vi "TestingThingsWithRobotSimulator.vi"() -> ()   [LabVIEW 2016]
uses:
  <vilib>/addons/control/pid/pid.llb/PID (DBL).vi
  <vilib>/addons/control/pid/NI_PID_pid.lvlib
panel:
  in  "Radius":dbl=200.0
  out "AngleVel":cluster{dbl, dbl}(graph)={199.99833333333333, 200.08337175954182}
  out "AnglePos":cluster{dbl, dbl}(graph)={199.99833333333333, 200.08337175954182}
  in  "Angular Constants":T1={"FF"=0.0085, "PID gains"={"P"=0.1, "I"=0.0, "D"=0.0}} {"PID gains"."D" format="%.5f"; "PID gains"."I" format="%.3f"; "PID gains"."P" format="%.3f"}
  out "Position":cluster{dbl, dbl}(graph)={199.99833333333333, 200.08337175954182}
  in  "Linear Constants":T1={"FF"=0.0085, "PID gains"={"P"=0.1, "I"=0.0, "D"=0.0}} {"PID gains"."D" format="%.5f"; "PID gains"."I" format="%.3f"; "PID gains"."P" format="%.3f"}
  out "Velocity":cluster{dbl, dbl}(graph)={-0.4999999999999858, -1.2779448924192138}
  in  "Distance":dbl=200.0
  in  "InitialVelocity":dbl
  in  "FinalVelocity":dbl
  in  "MaxVelocity":dbl=100.0
  in  "MaxAccel":dbl=75.0
  out "XY Graph":cluster{"X":dbl, "Y":dbl}[](graph)=[{"X"=200.08337175954182, "Y"=0.0}, {"X"=200.1089306573902, "Y"=0.0}, {"X"=200.10424441075094, "Y"=0.0}, {"X"=200.07099450505171, "Y"=0.0}, {"X"=200.00796286290563, "Y"=0.0}, {"X"=199.91051996431216, "Y"=0.0}, {"X"=199.78620155656287, "Y"=0.0}, {"X"=199.63192039247025, "Y"=0.0}, {"X"=199.44775349014458, "Y"=0.0}, {"X"=199.2445038727529, "Y"=0.0}, {"X"=199.00183461595887, "Y"=0.0}, {"X"=198.71497272839522, "Y"=0.0}, {"X"=198.41034772868528, "Y"=0.0}, {"X"=198.0759403876277, "Y"=0.0}, {"X"=197.73014814269519, "Y"=0.0}, {"X"=197.3171109110234, "Y"=0.0}, {"X"=196.8925644257071, "Y"=0.0}, {"X"=196.4385930075795, "Y"=0.0}, {"X"=195.9796929794355, "Y"=0.0}, {"X"=195.46712720086722, "Y"=0.0}, {"X"=194.89548304690467, "Y"=0.0}, {"X"=194.31956118281, "Y"=0.0}, {"X"=193.71392036197386, "Y"=0.0}, {"X"=193.07896301932513, "Y"=0.0}, {"X"=192.41522954143292, "Y"=0.0}, {"X"=191.7234038195058, "Y"=0.0}, {"X"=191.04025749483898, "Y"=0.0}, {"X"=190.29228445105284, "Y"=0.0}, {"X"=189.51289102295777, "Y"=0.0}, {"X"=188.66003856393252, "Y"=0.0}, {"X"=187.81626679449843, "Y"=0.0}, {"X"=186.94243421709916, "Y"=0.0}, {"X"=186.03850036846163, "Y"=0.0}, {"X"=185.10441535298747, "Y"=0.0}, {"X"=184.14012122839858, "Y"=0.0}, {"X"=183.1455552843998, "Y"=0.0}, {"X"=182.12065585459328, "Y"=0.0}, {"X"=181.06537132419885, "Y"=0.0}, {"X"=179.97967294093488, "Y"=0.0}, {"X"=178.8635718667005, "Y"=0.0}, {"X"=177.71714058083234, "Y"=0.0}, {"X"=176.54053821600394, "Y"=0.0}, {"X"=175.33403863100364, "Y"=0.0}, {"X"=174.0980589646555, "Y"=0.0}, {"X"=172.83318505393913, "Y"=0.0}, {"X"=171.5401884494904, "Y"=0.0}, {"X"=170.28603591065794, "Y"=0.0}, {"X"=168.86588931496718, "Y"=0.0}, {"X"=167.4837907214045, "Y"=0.0}, {"X"=166.14480489378158, "Y"=0.0}]
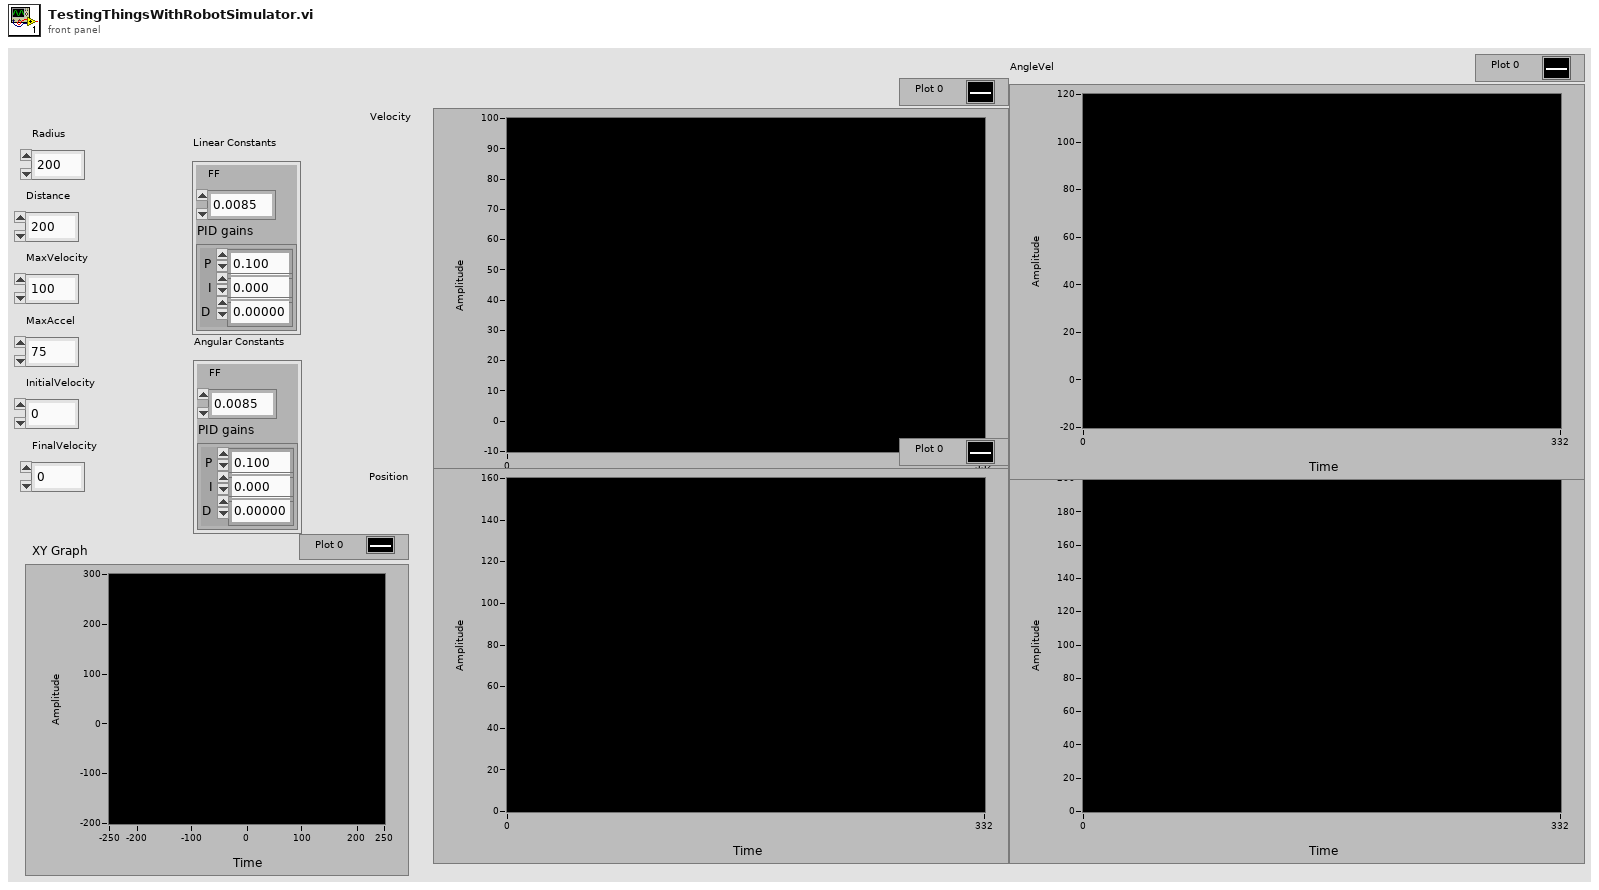
[diagram p1: front panel]
types:
  T1 = cluster{"FF":dbl, "PID gains":cluster{"P":dbl, "I":dbl, "D":dbl}}
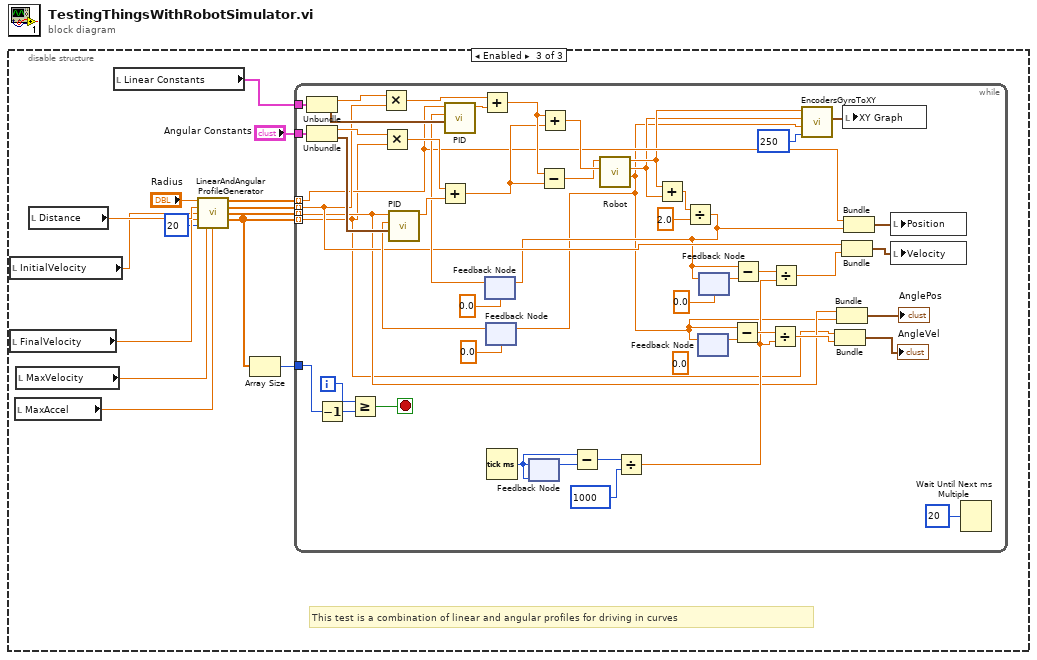
[diagram p0: block diagram]
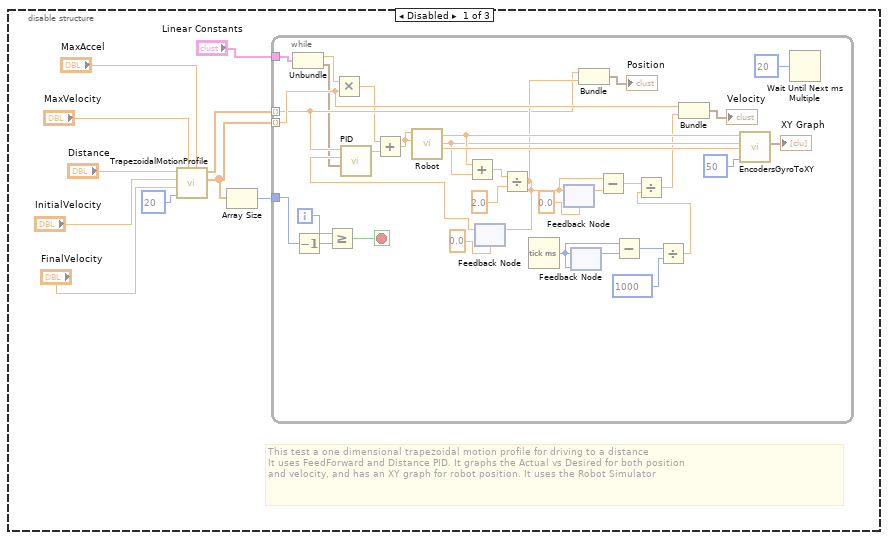
[diagram p2: hidden frame]
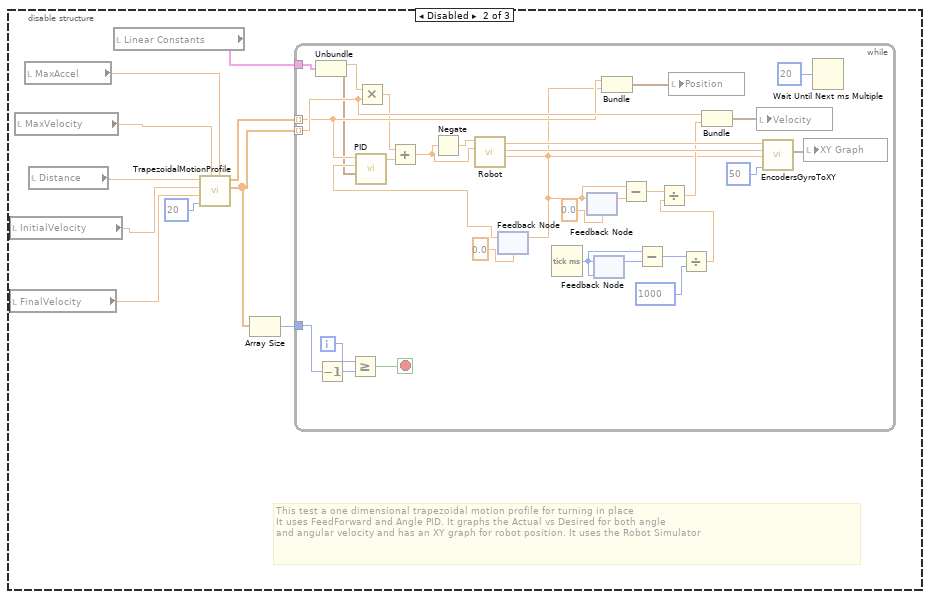
[diagram p3: hidden frame]
diagram:
  n1 = disable-structure shown="Enabled" {
    frame Disabled {
      # "This test a one dimensional trapezoidal motion profile for driving to a distance\nIt uses FeedForward and Distance PID. It graphs the Actual vs Desired for both position\nand velocity, and has an XY graph for robot position. It uses the Robot Simulator"
      n2 = call "TrapezoidalMotionProfile.vi"("MaxAccel"="MaxAccel", "MaxVelocity"="MaxVelocity", "dt"=u32 20, "FinalVelocity"="FinalVelocity", "InitialVelocity"="InitialVelocity", "Distance"="Distance") -> ("Vel"=w3:dbl[], "Pos"=w4:dbl[])  [unwired: 2 in, 2 out]
      n3 = Array Size(array=w3) -> (size(s)=w2:i32)
      n4 = while {
        tunnel: w4 -> [w15] mode=indexing
        tunnel: w3 -> [w20] mode=indexing
        tunnel: w2 -> [w32]
        tunnel: "Linear Constants" -> [w31]
        i -> [w35]
        stop <- w34 stop-if-true
        n5 = Unbundle(w31) -> ("FF"=w30:dbl, "PID gains"=w14:cluster{"P":dbl, "I":dbl, "D":dbl})
        n6 = Decrement(x=w32) -> (x-1=w33:i32)
        n7 = Greater Or Equal?(x=w35, y=w33) -> (x >= y?=w34:bool)
        n8 = Multiply(x=w30, y=w20) -> (x*y=w12:dbl)
        n9 = feedback #1(0.0) -> (w16:dbl)
        n10 = call-poly <vilib>:"PID.vi"("PID gains"=w14, "process variable"=w16, "setpoint"=w15) -> ("output"=w13:dbl)  [unwired: 7 in, 1 out]
        n11 = Add(x=w12, y=w13) -> (x+y=w11:dbl)
        n12 = call "Robot.vi"("Right Value"=w11, "Left Value"=w11) -> ("Angle"=w44:dbl, "Right Distance"=w39:dbl, "Left Distance"=w40:dbl)  [unwired: 7 in]
        n13 = Add(x=w40, y=w39) -> (x+y=w38:dbl)
        n14 = Divide(x=w38, y=2.0) -> (x/y=w17:dbl)
        n15 = feedback-in #1(w17) -> ()
        n16 = Tick Count (ms)() -> (millisecond timer value=w25:u32)
        n17 = feedback-in #2(w17) -> ()
        n18 = feedback #2(0.0) -> (w29:dbl)
        n19 = feedback #3(w25) -> (w26:u32)
        n20 = feedback-in #3(w25) -> ()
        n21 = Bundle(w15, w17) -> (→"Position":cluster{dbl, dbl})  [unwired: 1 in]
        n22 = Subtract(x=w17, y=w29) -> (x-y=w27:dbl)
        n23 = Subtract(x=w25, y=w26) -> (x-y=w24:u32)
        n24 = Divide(x=w24, y=u32 1000) -> (x/y=w22:dbl)
        n25 = Divide(x=w27, y=w22) -> (x/y=w21:dbl)
        n26 = Bundle(w20, w21) -> (→"Velocity":cluster{dbl, dbl})  [unwired: 1 in]
        n27 = call "EncodersGyroToXY.vi"("Locations to keep"=u32 50, "Angle (degrees)"=w44, "Right Distance"=w39, "Left Distance"=w40) -> ("XY Graph"=→"XY Graph":cluster{"X":dbl, "Y":dbl}[])  [unwired: 6 in, 1 out]
        n28 = Wait Until Next ms Multiple(millisecond multiple=u32 20 ("milliseconds to wait")) -> ()  [unwired: 1 out]
      }
    }
    frame Disabled {
      # "This test a one dimensional trapezoidal motion profile for turning in place\nIt uses FeedForward and Angle PID. It graphs the Actual vs Desired for both angle\nand angular velocity and has an XY graph for robot position. It uses the Robot Simulator"
      n29 = local read "InitialVelocity"() -> (w47:dbl)
      n30 = local read "FinalVelocity"() -> (w46:dbl)
      n31 = local read "MaxVelocity"() -> (w49:dbl)
      n32 = local read "MaxAccel"() -> (w50:dbl)
      n33 = local read "Distance"() -> (w48:dbl)
      n34 = local read "Linear Constants"() -> (w45:T1)
      n35 = call "TrapezoidalMotionProfile.vi"("MaxAccel"=w50, "MaxVelocity"=w49, "dt"=u32 20, "FinalVelocity"=w46, "InitialVelocity"=w47, "Distance"=w48) -> ("Vel"=w52:dbl[], "Pos"=w53:dbl[])  [unwired: 2 in, 2 out]
      n36 = Array Size(array=w52) -> (size(s)=w51:i32)
      n37 = while {
        tunnel: w53 -> [w64] mode=indexing
        tunnel: w52 -> [w66] mode=indexing
        tunnel: w51 -> [w78]
        tunnel: w45 -> [w77]
        i -> [w81]
        stop <- w80 stop-if-true
        n38 = Unbundle(w77) -> ("FF"=w76:dbl, "PID gains"=w63:cluster{"P":dbl, "I":dbl, "D":dbl})
        n39 = Decrement(x=w78) -> (x-1=w79:i32)
        n40 = Greater Or Equal?(x=w81, y=w79) -> (x >= y?=w80:bool)
        n41 = Multiply(x=w76, y=w66) -> (x*y=w61:dbl)
        n42 = feedback #4(0.0) -> (w65:dbl)
        n43 = call-poly <vilib>:"PID.vi"("PID gains"=w63, "process variable"=w65, "setpoint"=w64) -> ("output"=w62:dbl)  [unwired: 7 in, 1 out]
        n44 = Add(x=w61, y=w62) -> (x+y=w56:dbl)
        n45 = Negate(x=w56) -> (-x=w57:dbl)
        n46 = call "Robot.vi"("Right Value"=w56, "Left Value"=w57) -> ("Angle"=w58:dbl, "Right Distance"=w83:dbl, "Left Distance"=w84:dbl)  [unwired: 7 in]
        n47 = feedback-in #4(w58) -> ()
        n48 = Tick Count (ms)() -> (millisecond timer value=w71:u32)
        n49 = feedback-in #5(w58) -> ()
        n50 = feedback #5(0.0) -> (w75:dbl)
        n51 = feedback #6(w71) -> (w72:u32)
        n52 = feedback-in #6(w71) -> ()
        n53 = Bundle(w64, "Angle"=w58) -> (w59:cluster{dbl, "Angle":dbl})  [unwired: 1 in]
        n54 = Subtract(x=w58, y=w75) -> (x-y=w73:dbl)
        n55 = Subtract(x=w71, y=w72) -> (x-y=w70:u32)
        n56 = local write "Position"(w59) -> ()
        n57 = Divide(x=w70, y=u32 1000) -> (x/y=w68:dbl)
        n58 = Divide(x=w73, y=w68) -> (x/y=w67:dbl)
        n59 = Bundle(w66, w67) -> (w60:cluster{dbl, dbl})  [unwired: 1 in]
        n60 = local write "Velocity"(w60) -> ()
        n61 = call "EncodersGyroToXY.vi"("Locations to keep"=u32 50, "Angle (degrees)"=w58, "Right Distance"=w83, "Left Distance"=w84) -> ("XY Graph"=w55:cluster{"X":dbl, "Y":dbl}[])  [unwired: 6 in, 1 out]
        n62 = local write "XY Graph"(w55) -> ()
        n63 = Wait Until Next ms Multiple(millisecond multiple=u32 20 ("milliseconds to wait")) -> ()  [unwired: 1 out]
      }
    }
    frame Enabled {
      # "This test is a combination of linear and angular profiles for driving in curves"
      n64 = local read "InitialVelocity"() -> (w96:dbl)
      n65 = local read "FinalVelocity"() -> (w95:dbl)
      n66 = local read "MaxAccel"() -> (w93:dbl)
      n67 = local read "MaxVelocity"() -> (w94:dbl)
      n68 = local read "Distance"() -> (w97:dbl)
      n69 = local read "Linear Constants"() -> (w99:T1)
      n70 = call "LinearAndAngularProfileGenerator.vi"("Radius"="Radius", "Theta"=w97, "InitialVelocity"=w96, "FinalVelocity"=w95, "dt"=u32 20, "MaxVelocity"=w94, "MaxAccel"=w93) -> ("Pos"=w90:dbl[], "Vel"=w89:dbl[], "AnglePos"=w88:dbl[], "AngularVel"=w87:dbl[])  [unwired: 4 in, 1 out]
      n71 = Array Size(array=w87) -> (size(s)=w100:i32)
      n72 = while {
        tunnel: w100 -> [w146]
        tunnel: w99 -> [w137]
        tunnel: "Angular Constants" -> [w136]
        tunnel: w90 -> [w113] mode=indexing
        tunnel: w89 -> [w115] mode=indexing
        tunnel: w88 -> [w109] mode=indexing
        tunnel: w87 -> [w108] mode=indexing
        i -> [w149]
        stop <- w148 stop-if-true
        (unwired) 0.0
        n73 = Unbundle(w137) -> ("FF"=w145:dbl, "PID gains"=w134:cluster{"P":dbl, "I":dbl, "D":dbl})
        n74 = Unbundle(w136) -> ("FF"=w135:dbl, "PID gains"=w133:cluster{"P":dbl, "I":dbl, "D":dbl})
        n75 = Decrement(x=w146) -> (x-1=w147:i32)
        n76 = Greater Or Equal?(x=w149, y=w147) -> (x >= y?=w148:bool)
        n77 = Multiply(x=w145, y=w115) -> (x*y=w130:dbl)
        n78 = Multiply(x=w135, y=w108) -> (x*y=w132:dbl)
        n79 = feedback #7(0.0) -> (w122:dbl)
        n80 = call-poly <vilib>:"PID.vi"("PID gains"=w134, "process variable"=w122, "setpoint"=w113) -> ("output"=w129:dbl)  [unwired: 7 in, 1 out]
        n81 = Add(x=w130, y=w129) -> (x+y=w127:dbl)
        n82 = feedback #8(0.0) -> (w120:dbl)
        n83 = call-poly <vilib>:"PID.vi"("PID gains"=w133, "process variable"=w120, "setpoint"=w109) -> ("output"=w131:dbl)  [unwired: 7 in, 1 out]
        n84 = Add(x=w132, y=w131) -> (x+y=w126:dbl)
        n85 = Tick Count (ms)() -> (millisecond timer value=w140:u32)
        n86 = feedback #9(w140) -> (w141:u32)
        n87 = feedback-in #9(w140) -> ()
        n88 = Subtract(x=w127, y=w126) -> (x-y=w125:dbl)
        n89 = Add(x=w127, y=w126) -> (x+y=w128:dbl)
        n90 = Subtract(x=w140, y=w141) -> (x-y=w139:u32)
        n91 = call "Robot.vi"("Right Value"=w128, "Left Value"=w125) -> ("Angle"=w101:dbl, "Right Distance"=w102:dbl, "Left Distance"=w103:dbl)  [unwired: 7 in]
        n92 = feedback-in #8(w101) -> ()
        n93 = Divide(x=w139, y=u32 1000) -> (x/y=w117:dbl)
        n94 = Add(x=w103, y=w102) -> (x+y=w124:dbl)
        n95 = Divide(x=w124, y=2.0) -> (x/y=w114:dbl)
        n96 = feedback-in #7(w114) -> ()
        n97 = feedback #10() -> (w118:dbl)  [unwired: 1 in]
        n98 = feedback-in #10(w101) -> ()
        n99 = feedback-in #11(w114) -> ()
        n100 = feedback #11(0.0) -> (w144:dbl)
        n101 = Subtract(x=w101, y=w118) -> (x-y=w119:dbl)
        n102 = Subtract(x=w114, y=w144) -> (x-y=w142:dbl)
        n103 = Divide(x=w119, y=w117) -> (x/y=w110:dbl)
        n104 = Divide(x=w142, y=w117) -> (x/y=w116:dbl)
        n105 = call "EncodersGyroToXY.vi"("Locations to keep"=u32 250, "Angle (degrees)"=w101, "Right Distance"=w102, "Left Distance"=w103) -> ("XY Graph"=w104:cluster{"X":dbl, "Y":dbl}[])  [unwired: 6 in, 1 out]
        n106 = Bundle(w108, w110) -> (→"AngleVel":cluster{dbl, dbl})  [unwired: 1 in]
        n107 = Bundle(w109, "Angle"=w101) -> (→"AnglePos":cluster{dbl, "Angle":dbl})  [unwired: 1 in]
        n108 = Bundle(w115, w116) -> (w111:cluster{dbl, dbl})  [unwired: 1 in]
        n109 = local write "XY Graph"(w104) -> ()
        n110 = Bundle(w113, w114) -> (w112:cluster{dbl, dbl})  [unwired: 1 in]
        n111 = local write "Position"(w112) -> ()
        n112 = local write "Velocity"(w111) -> ()
        n113 = Wait Until Next ms Multiple(millisecond multiple=u32 20 ("milliseconds to wait")) -> ()  [unwired: 1 out]
      }
    }
  }
